vi "Get Step By Index.vi"(8 "error in (no error)":errorcluster, 10 "Index":i32, 11 "Recipe in":refnum<class "Recipe.lvclass">) -> (0 "error out":errorcluster, 2 "Recipe Step":refnum<class "Recipe Step.lvclass">, 3 "Recipe out":refnum<class "Recipe.lvclass">)   [LabVIEW 2024, in "Recipe.lvclass"]
uses:
  Recipe.lvclass
  Recipe.lvclass/Recipe.ctl
  Recipe Step/Recipe Step.lvclass
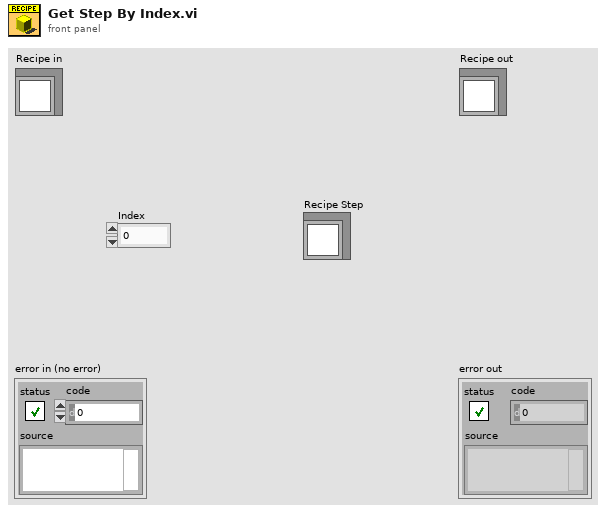
[diagram p1: front panel]
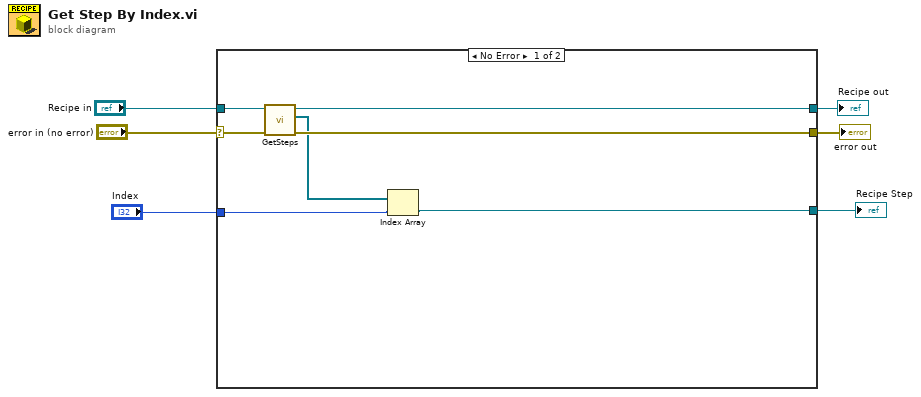
[diagram p0: block diagram]
diagram:
  n1 = case shown="No Error" "error in (no error)" {
    selector: "error in (no error)" -> [w13 w15]
    tunnel: [w12 w15] -> w5
    tunnel: [w10 w14] -> w3
    tunnel: "Recipe in" -> [w11 w14]
    tunnel: "Index" -> [w8 _]
    tunnel: [w7 _] -> w1
    frame No Error {
      n2 = call-dynamic "GetSteps.vi"("Error In"=w13, "reference in"=w11) -> ("Error Out"=w12:errorcluster, "Steps"=w9:refnum<class "Recipe Step.lvclass">[], "reference out"=w10:refnum<class "Recipe.lvclass">)  [unwired: 7 in]
      n3 = Index Array(array=w9, index=w8) -> (element=w7:refnum<class "Recipe Step.lvclass">)
    }
    frame Error {
    }
  }
  "error out" <- w5
  "Recipe out" <- w3
  "Recipe Step" <- w1
